vi "TL27_Get_Raw_Fault_Snapshot.vi"(0 "GEA2 Reference In":refnum<k24>, 5 "GEA Inputs":T3={"Source"=228, "Destination"=35} {"Destination" format="%.0x"; "Source" format="%.0x"}, 7 "Standalone":bool, 11 "Error In":errorcluster) -> (4 "GEA2 Reference Out":refnum<k24>, 8 "Array":T1(array[cluster]), 15 "Error Out":errorcluster)   [LabVIEW 2016]
uses:
  Common/LabVIEW GEA2 Toolkit/LabVIEW_GEA2_Toolkit.lvlibp/type defs/Source_Destination.ctl
  Q:/Common/DLLs/GEA3/GeaCommunication.dll
  Common/DLLs/GEA3/GeaCommunication.dll
  Common/LabVIEW GEA2 Toolkit/LabVIEW_GEA2_Toolkit.lvlibp/type defs/ERD Read Data In.ctl
  Common/LabVIEW GEA2 Toolkit/LabVIEW_GEA2_Toolkit.lvlibp/type defs/Data Type.ctl
  Common/LabVIEW GEA2 Toolkit/LabVIEW_GEA2_Toolkit.lvlibp
panel:
  in  "input cluster":T2
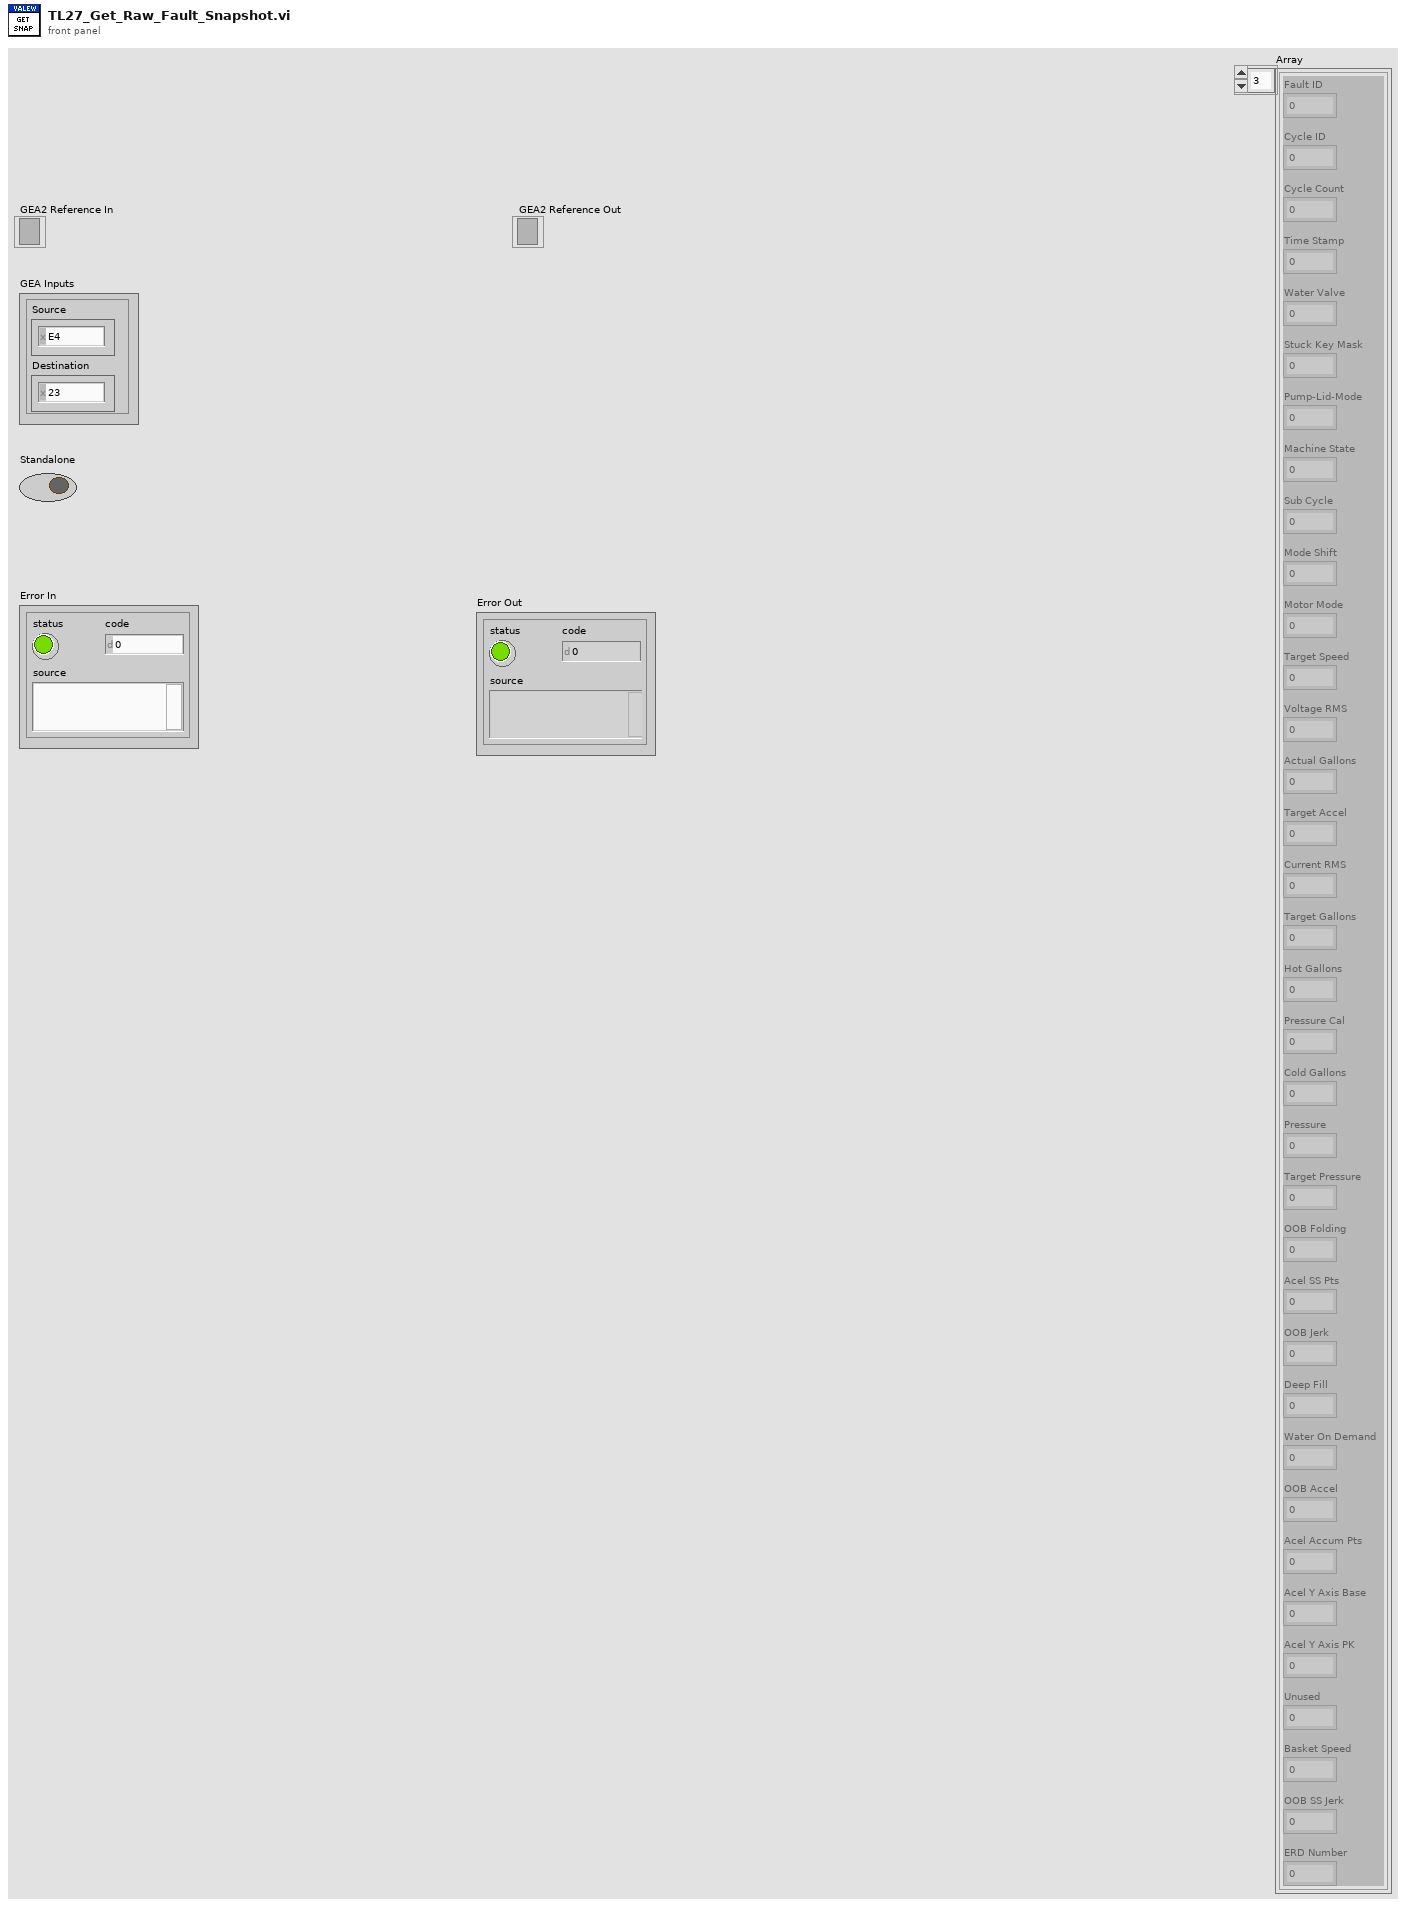
[diagram p1: front panel]
types:
  T1 = cluster{"Fault ID":u16, "Cycle ID":u8, "Cycle Count":u32, "Time Stamp":u32, "Water Valve":u8, "Stuck Key Mask":u64, "Pump-Lid-Mode":u8, "Machine State":u8, "Sub Cycle":u8, "Mode Shift":u8, "Motor Mode":u8, "Target Speed":i16, "Voltage RMS":u16, "Actual Gallons":u16, "Target Accel":u16, "Current RMS":u16, "Target Gallons":u16, "Hot Gallons":u16, "Pressure Cal":u32, "Cold Gallons":u16, "Pressure ":u32, "Target Pressure":u32, "OOB Folding":i32, "Acel SS Pts":u8, "OOB Jerk":i32, "Deep Fill":u8, "Water On Demand":u8, "OOB Accel":i32, "Acel Accum Pts":u8, "Acel Y Axis Base":i16, "Acel Y Axis PK":i16, "Unused":u8, "Basket Speed":u16, "OOB SS Jerk":i32, "ERD Number":u64}[]
  T2 = cluster{"Fault ID":u16, "Cycle ID":u8, "Cycle Count":u32, "Time Stamp":u32, "Water Valve":u8, "Stuck Key Mask":u64, "Pump-Lid-Mode":u8, "Machine State":u8, "Sub Cycle":u8, "Mode Shift":u8, "Motor Mode":u8, "Target Speed":i16, "Voltage RMS":u16, "Actual Gallons":u16, "Target Accel":u16, "Current RMS":u16, "Target Gallons":u16, "Hot Gallons":u16, "Pressure Cal":u32, "Cold Gallons":u16, "Pressure ":u32, "Target Pressure":u32, "OOB Folding":i32, "Acel SS Pts":u8, "OOB Jerk":i32, "Deep Fill":u8, "Water On Demand":u8, "OOB Accel":i32, "Acel Accum Pts":u8, "Acel Y Axis Base":i16, "Acel Y Axis PK":i16, "Unused":u8, "Basket Speed":u16, "OOB SS Jerk":i32, "ERD Number":u64}
  T3 = typedef "LabVIEW_GEA2_Toolkit.lvlibp/Source_Destination.ctl" = cluster{"Source":u8, "Destination":u8}
  T4 = typedef "LabVIEW_GEA2_Toolkit.lvlibp/ERD Read Data In.ctl" = cluster{"ERD Number":u16, "Data Type":T5}
  T5 = typedef "LabVIEW_GEA2_Toolkit.lvlibp/Data Type.ctl" = enum16{"string", "boolean", "uint8_t", "uint16_t", "uint32_t", "uint64_t", "int8_t", "int16_t", "int32_t", "int64_t"}
  T6 = typedef "LabVIEW_GEA2_Toolkit.lvlibp/ERD Read Data Out.ctl" = cluster{"ERD Number":u16, "Data":string}
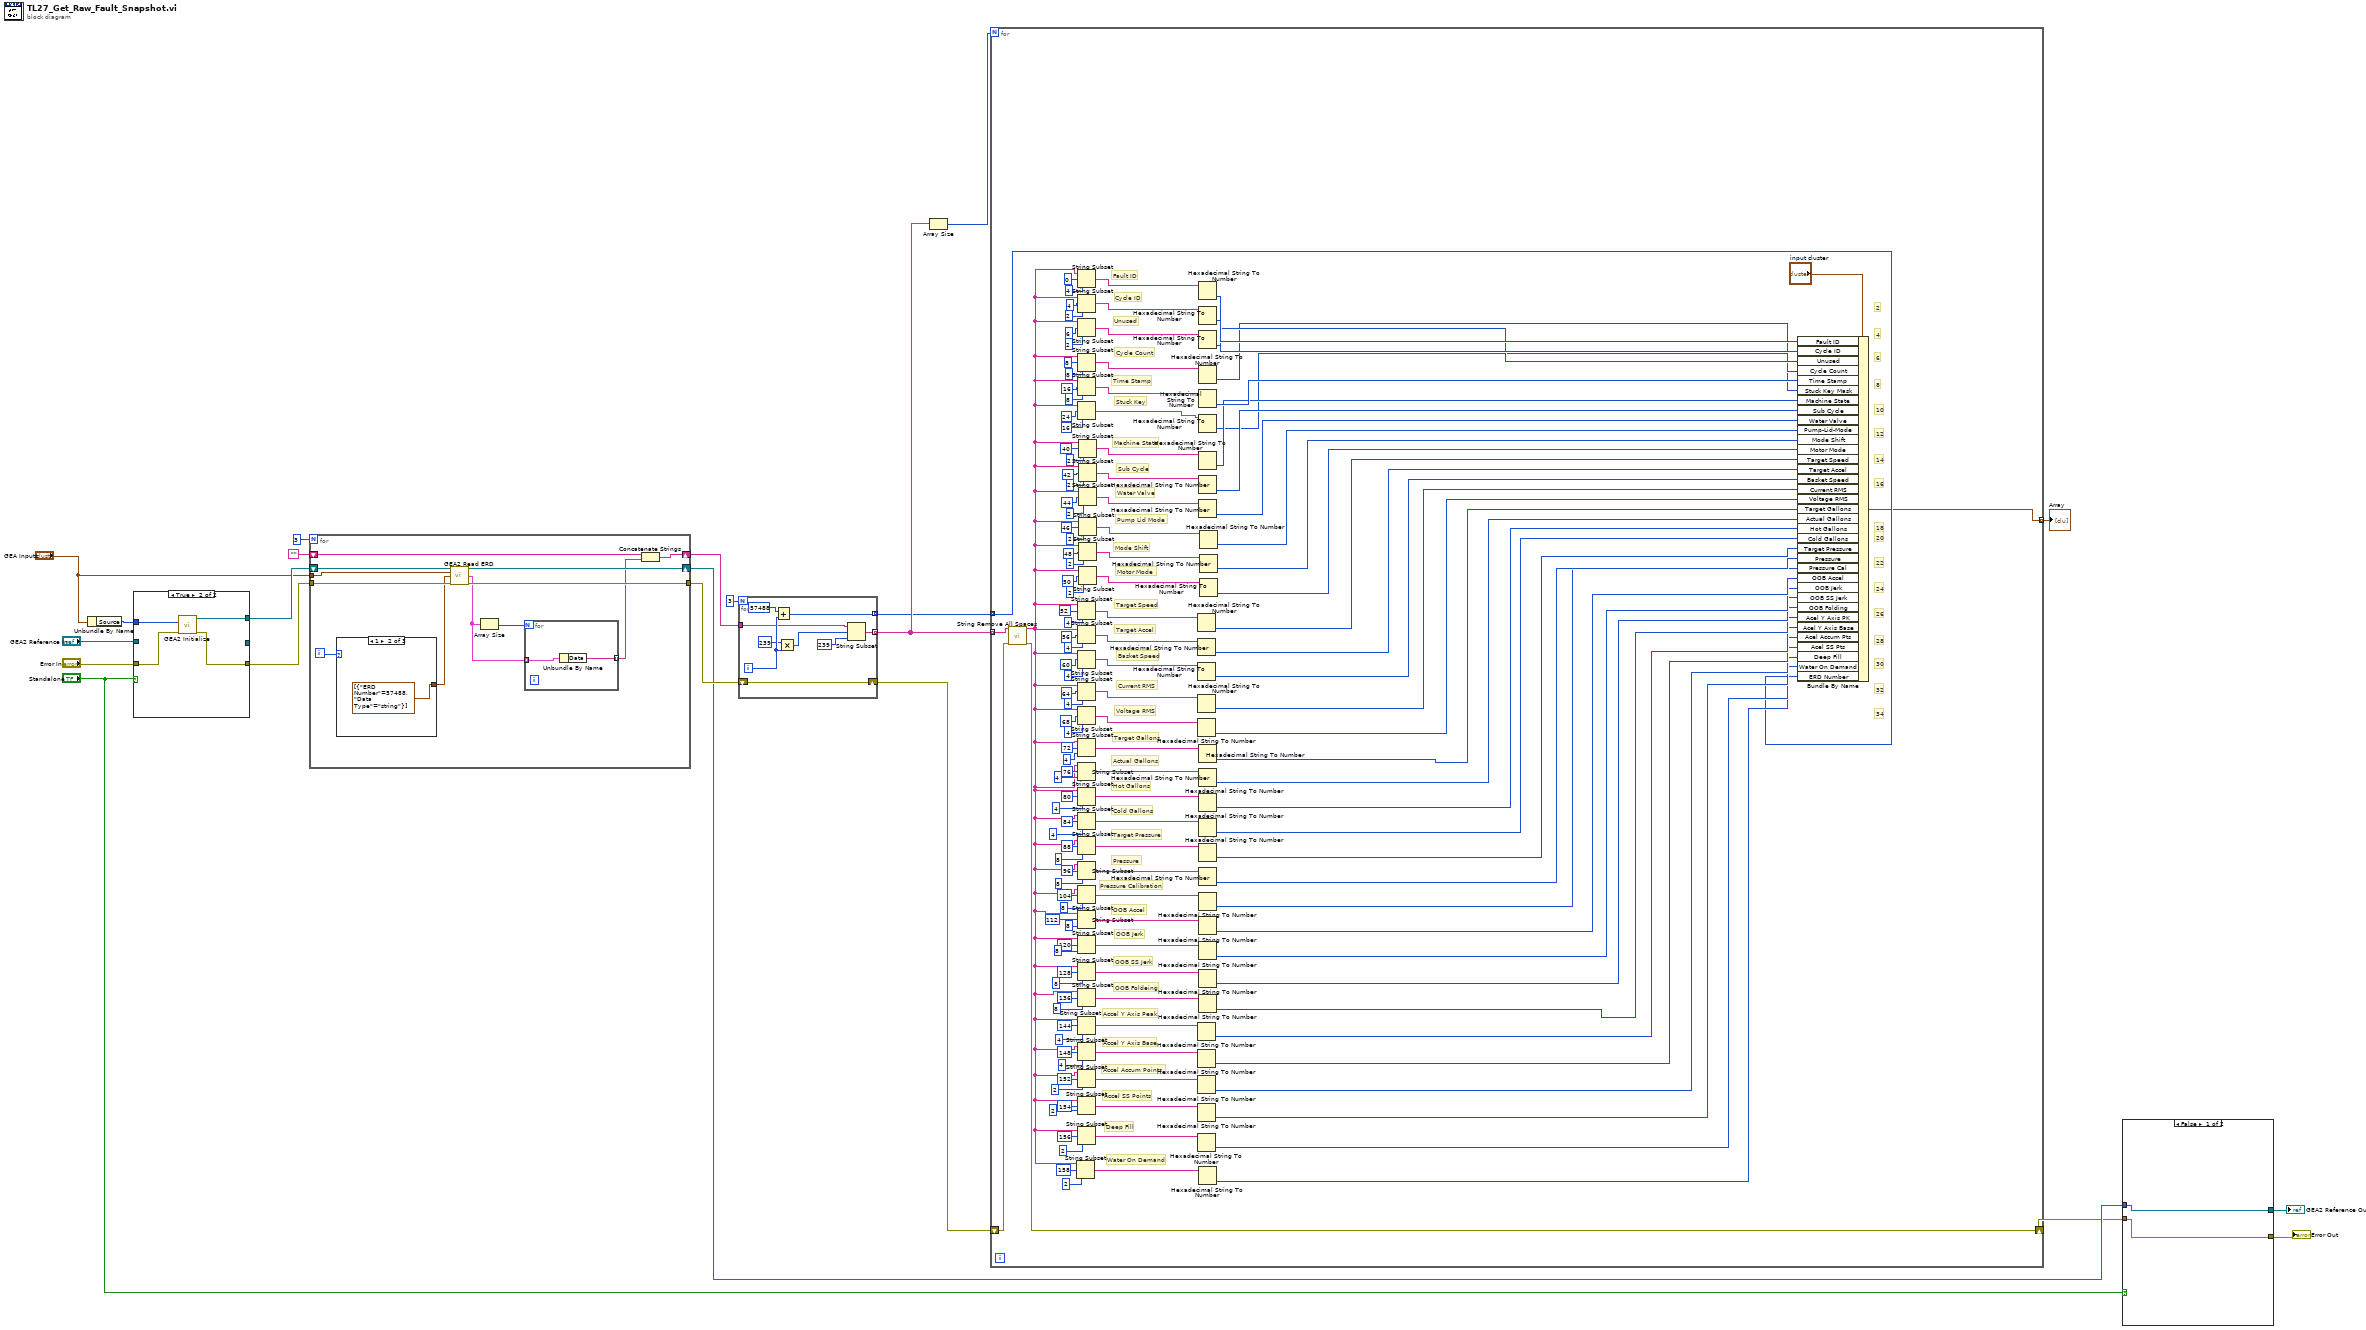
[diagram p0: block diagram]
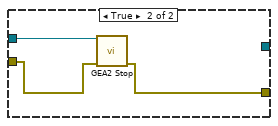
[diagram p2: hidden frame]
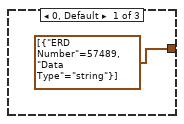
[diagram p4: hidden frame]
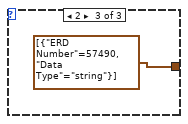
[diagram p5: hidden frame]
diagram:
  n1 = Unbundle By Name("GEA Inputs") -> ("Source"=w15:u8)
  n2 = case shown="True" "Standalone" {
    tunnel: [w23 w24] -> w12
    tunnel: "Error In" -> [w23 w25]
    tunnel: [w22 _] -> _
    tunnel: "GEA2 Reference In" -> [w22 _]
    tunnel: w15 -> [_ w27]
    tunnel: [_ w26] -> w14
    frame False {
    }
    frame True {
      n3 = call "GEA2 Initialize.vi"("Source Address"=w27, "error in"=w25) -> ("GEA2 Reference Out"=w26:refnum<k24>, "error out"=w24:errorcluster)  [unwired: 11 in, 1 out]
    }
  }
  n4 = for {
    N: 3 -> [_]
    shift-right: [w38] -> w1
    shift-left: "" -> [w37]
    shift-right: [w34] -> w10
    shift-left: w14 -> [w35]
    tunnel: w12 -> [w33]
    tunnel: [w32] -> w11
    tunnel: "GEA Inputs" -> [w30]
    i -> [w36]
    n5 = case shown="1" w36 {
      tunnel: [T4[] [{"ERD Number"=57489, "Data Type"=enum."string"}] ("Read ERD List") T4[] [{"ERD Number"=57488, "Data Type"=enum."string"}] ("Read ERD List") T4[] [{"ERD Number"=57490, "Data Type"=enum."string"}] ("Read ERD List")] -> w31
      frame 0, Default {
      }
      frame 1 {
      }
      frame 2 {
      }
    }
    n6 = call "GEA2 Read ERD.vi"("GEA2 Reference In"=w35, "GEA Inputs"=w30, "Read ERD List"=w31, "Error In"=w33) -> ("GEA2 Reference Out"=w34:refnum<k24>, "ERD Data Out"=w28:T6[], "Error Out"=w32:errorcluster)  [unwired: 8 in, 1 out]
    n7 = Array Size(array=w28) -> (size(s)=w39:i32)
    n8 = for {
      N: w39 -> [_]
      tunnel: [w41] -> w29 mode=indexing
      tunnel: w28 -> [w40] mode=indexing
      n9 = Unbundle By Name(w40) -> ("Data"=w41:string)
    }
    n10 = Concatenate Strings(w37, w29) -> (w38:string)
  }
  n11 = for {
    N: 3 -> [_]
    tunnel: [w51] -> w3 mode=indexing
    shift-right: [w50] -> w6
    shift-left: w11 -> [w50]
    tunnel: [w45] -> w19 mode=indexing
    tunnel: w1 -> [w46]
    i -> [w49]
    n12 = Add(x=57488, y=w49) -> (x+y=w51:i32)
    n13 = Multiply(x=239, y=w49) -> (x*y=w47:i32)
    n14 = String Subset(string=w46, offset (0)=w47, length (rest)=239 ("length (rest)")) -> (substring=w45:string)
  }
  n15 = Array Size(array=w19) -> (size(s)=w21:i32)
  n16 = for {
    N: w21 -> [_]
    tunnel: w19 -> [w61] mode=indexing
    shift-right: [w59] -> w5
    shift-left: w6 -> [w60]
    tunnel: w3 -> [w58] mode=indexing
    tunnel: [w56] -> w2 mode=indexing
    # "Stuck Key"
    # "Deep Fill"
    # "Accel SS Points"
    # "Accel Accum Points"
    # "Accel Y Axis Base"
    # "OOB Foldeing"
    # "OOB SS Jerk"
    # "OOB Accel"
    # "Pressure"
    # "Cold Gallons"
    # "Actual Gallons"
    # "Voltage RMS"
    # "Basket Speed"
    # "Target Speed"
    # "Mode Shift"
    # "Water Valve"
    # "Machine State"
    # "Time Stamp"
    # "Unused"
    # "Fault ID"
    # "34"
    # "32"
    # "30"
    # "28"
    # "26"
    # "24"
    # "22"
    # "20"
    # "18"
    # "16"
    # "14"
    # "12"
    # "10"
    # "8"
    # "6"
    # "4"
    # "2"
    # "Water On Demand"
    # "Accel Y Axis Peak"
    # "OOB Jerk"
    # "Pressure Calibration"
    # "Target Pressure"
    # "Hot Gallons"
    # "Target Gallons"
    # "Current RMS"
    # "Target Accel"
    # "Motor Mode"
    # "Pump Lid Mode"
    # "Sub Cycle"
    # "Cycle Count"
    # "Cycle ID"
    n17 = call "String Remove All Spaces.vi"("Input String"=w61, "error in (no error)"=w60) -> ("Spaces Removed"=w62:string, "error out"=w59:errorcluster)  [unwired: 12 in]
    n18 = String Subset(string=w62, offset (0)=158, length (rest)=2 ("length (rest)")) -> (substring=w137:string)
    n19 = String Subset(string=w62, offset (0)=52, length (rest)=4 ("length (rest)")) -> (substring=w105:string)
    n20 = String Subset(string=w62, offset (0)=56, length (rest)=4 ("length (rest)")) -> (substring=w104:string)
    n21 = String Subset(string=w62, offset (0)=60, length (rest)=4 ("length (rest)")) -> (substring=w103:string)
    n22 = String Subset(string=w62, offset (0)=64, length (rest)=4 ("length (rest)")) -> (substring=w98:string)
    n23 = String Subset(string=w62, offset (0)=68, length (rest)=4 ("length (rest)")) -> (substring=w97:string)
    n24 = String Subset(string=w62, offset (0)=0, length (rest)=4 ("length (rest)")) -> (substring=w158:string)
    n25 = String Subset(string=w62, offset (0)=4, length (rest)=2 ("length (rest)")) -> (substring=w157:string)
    n26 = String Subset(string=w62, offset (0)=6, length (rest)=2 ("length (rest)")) -> (substring=w156:string)
    n27 = String Subset(string=w62, offset (0)=8, length (rest)=8 ("length (rest)")) -> (substring=w130:string)
    n28 = String Subset(string=w62, offset (0)=16, length (rest)=8 ("length (rest)")) -> (substring=w129:string)
    n29 = String Subset(string=w62, offset (0)=24, length (rest)=16 ("length (rest)")) -> (substring=w55:string)
    n30 = String Subset(string=w62, offset (0)=72, length (rest)=4 ("length (rest)")) -> (substring=w155:string)
    n31 = String Subset(string=w62, offset (0)=76, length (rest)=4 ("length (rest)")) -> (substring=w154:string)
    n32 = String Subset(string=w62, offset (0)=80, length (rest)=4 ("length (rest)")) -> (substring=w153:string)
    n33 = String Subset(string=w62, offset (0)=84, length (rest)=4 ("length (rest)")) -> (substring=w152:string)
    n34 = String Subset(string=w62, offset (0)=88, length (rest)=8 ("length (rest)")) -> (substring=w151:string)
    n35 = String Subset(string=w62, offset (0)=96, length (rest)=8 ("length (rest)")) -> (substring=w150:string)
    n36 = String Subset(string=w62, offset (0)=104, length (rest)=8 ("length (rest)")) -> (substring=w149:string)
    n37 = String Subset(string=w62, offset (0)=112, length (rest)=8 ("length (rest)")) -> (substring=w148:string)
    n38 = String Subset(string=w62, offset (0)=120, length (rest)=8 ("length (rest)")) -> (substring=w147:string)
    n39 = String Subset(string=w62, offset (0)=128, length (rest)=8 ("length (rest)")) -> (substring=w146:string)
    n40 = String Subset(string=w62, offset (0)=136, length (rest)=8 ("length (rest)")) -> (substring=w145:string)
    n41 = String Subset(string=w62, offset (0)=144, length (rest)=4 ("length (rest)")) -> (substring=w144:string)
    n42 = String Subset(string=w62, offset (0)=148, length (rest)=4 ("length (rest)")) -> (substring=w143:string)
    n43 = String Subset(string=w62, offset (0)=152, length (rest)=2 ("length (rest)")) -> (substring=w142:string)
    n44 = String Subset(string=w62, offset (0)=154, length (rest)=2 ("length (rest)")) -> (substring=w141:string)
    n45 = String Subset(string=w62, offset (0)=156, length (rest)=2 ("length (rest)")) -> (substring=w140:string)
    n46 = String Subset(string=w62, offset (0)=40, length (rest)=2 ("length (rest)")) -> (substring=w122:string)
    n47 = String Subset(string=w62, offset (0)=42, length (rest)=2 ("length (rest)")) -> (substring=w121:string)
    n48 = String Subset(string=w62, offset (0)=44, length (rest)=2 ("length (rest)")) -> (substring=w120:string)
    n49 = String Subset(string=w62, offset (0)=46, length (rest)=2 ("length (rest)")) -> (substring=w113:string)
    n50 = String Subset(string=w62, offset (0)=48, length (rest)=2 ("length (rest)")) -> (substring=w112:string)
    n51 = String Subset(string=w62, offset (0)=50, length (rest)=2 ("length (rest)")) -> (substring=w63:string)
    n52 = Hexadecimal String To Number(string=w105) -> (number=w85:u32)  [unwired: 2 in, 1 out]
    n53 = Hexadecimal String To Number(string=w104) -> (number=w84:u32)  [unwired: 2 in, 1 out]
    n54 = Hexadecimal String To Number(string=w103) -> (number=w83:u32)  [unwired: 2 in, 1 out]
    n55 = Hexadecimal String To Number(string=w98) -> (number=w82:u32)  [unwired: 2 in, 1 out]
    n56 = Hexadecimal String To Number(string=w97) -> (number=w81:u32)  [unwired: 2 in, 1 out]
    n57 = Hexadecimal String To Number(string=w144) -> (number=w69:u32)  [unwired: 2 in, 1 out]
    n58 = Hexadecimal String To Number(string=w143) -> (number=w68:u32)  [unwired: 2 in, 1 out]
    n59 = Hexadecimal String To Number(string=w142) -> (number=w67:u32)  [unwired: 2 in, 1 out]
    n60 = Hexadecimal String To Number(string=w141) -> (number=w66:u32)  [unwired: 2 in, 1 out]
    n61 = Hexadecimal String To Number(string=w140) -> (number=w65:u32)  [unwired: 2 in, 1 out]
    n62 = Hexadecimal String To Number(string=w158) -> (number=w96:u32)  [unwired: 2 in, 1 out]
    n63 = Hexadecimal String To Number(string=w157) -> (number=w95:u32)  [unwired: 2 in, 1 out]
    n64 = Hexadecimal String To Number(string=w156) -> (number=w94:u32)  [unwired: 2 in, 1 out]
    n65 = Hexadecimal String To Number(string=w130) -> (number=w93:u32)  [unwired: 2 in, 1 out]
    n66 = Hexadecimal String To Number(string=w129) -> (number=w92:u32)  [unwired: 2 in, 1 out]
    n67 = Hexadecimal String To Number(string=w55) -> (number=w54:u32)  [unwired: 2 in, 1 out]
    n68 = Hexadecimal String To Number(string=w155) -> (number=w80:u32)  [unwired: 2 in, 1 out]
    n69 = Hexadecimal String To Number(string=w154) -> (number=w79:u32)  [unwired: 2 in, 1 out]
    n70 = Hexadecimal String To Number(string=w153) -> (number=w78:u32)  [unwired: 2 in, 1 out]
    n71 = Hexadecimal String To Number(string=w152) -> (number=w77:u32)  [unwired: 2 in, 1 out]
    n72 = Hexadecimal String To Number(string=w151) -> (number=w76:u32)  [unwired: 2 in, 1 out]
    n73 = Hexadecimal String To Number(string=w150) -> (number=w75:u32)  [unwired: 2 in, 1 out]
    n74 = Hexadecimal String To Number(string=w149) -> (number=w74:u32)  [unwired: 2 in, 1 out]
    n75 = Hexadecimal String To Number(string=w148) -> (number=w73:u32)  [unwired: 2 in, 1 out]
    n76 = Hexadecimal String To Number(string=w147) -> (number=w72:u32)  [unwired: 2 in, 1 out]
    n77 = Hexadecimal String To Number(string=w146) -> (number=w71:u32)  [unwired: 2 in, 1 out]
    n78 = Hexadecimal String To Number(string=w145) -> (number=w70:u32)  [unwired: 2 in, 1 out]
    n79 = Hexadecimal String To Number(string=w137) -> (number=w64:u32)  [unwired: 2 in, 1 out]
    n80 = Hexadecimal String To Number(string=w122) -> (number=w91:u32)  [unwired: 2 in, 1 out]
    n81 = Hexadecimal String To Number(string=w121) -> (number=w90:u32)  [unwired: 2 in, 1 out]
    n82 = Hexadecimal String To Number(string=w120) -> (number=w89:u32)  [unwired: 2 in, 1 out]
    n83 = Hexadecimal String To Number(string=w113) -> (number=w88:u32)  [unwired: 2 in, 1 out]
    n84 = Hexadecimal String To Number(string=w112) -> (number=w87:u32)  [unwired: 2 in, 1 out]
    n85 = Hexadecimal String To Number(string=w63) -> (number=w86:u32)  [unwired: 2 in, 1 out]
    n86 = Bundle By Name(cluster="input cluster", "Fault ID"=w96, "Cycle ID"=w95, "Unused"=w94, "Cycle Count"=w93, "Time Stamp"=w92, "Stuck Key Mask"=w54, "Machine State"=w91, "Sub Cycle"=w90, "Water Valve"=w89, "Pump-Lid-Mode"=w88, "Mode Shift"=w87, "Motor Mode"=w86, "Target Speed"=w85, "Target Accel"=w84, "Basket Speed"=w83, "Current RMS"=w82, "Voltage RMS"=w81, "Target Gallons"=w80, "Actual Gallons"=w79, "Hot Gallons"=w78, "Cold Gallons"=w77, "Target Pressure"=w76, "Pressure"=w75, "Pressure Cal"=w74, "OOB Accel"=w73, "OOB Jerk"=w72, "OOB SS Jerk"=w71, "OOB Folding"=w70, "Acel Y Axis PK"=w69, "Acel Y Axis Base"=w68, "Acel Accum Pts"=w67, "Acel SS Pts"=w66, "Deep Fill"=w65, "Water On Demand"=w64, "ERD Number"=w58) -> (w56:T2)
  }
  "Array" <- w2
  n87 = case shown="False" "Standalone" {
    tunnel: w10 -> [w198 w201]
    tunnel: [w198 _] -> w9
    tunnel: w5 -> [w197 w200]
    tunnel: [w197 w199] -> w4
    frame False {
    }
    frame True {
      n88 = call "GEA2 Stop.vi"("GEA2 Reference In"=w201, "Error In"=w200) -> ("Error Out"=w199:errorcluster)  [unwired: 13 in]
    }
  }
  "GEA2 Reference Out" <- w9
  "Error Out" <- w4
